vi "HideVIWindow.vi"(8 "ErrorIn":errorcluster, 11 "VIPath":path) -> (0 "ErrorOut":errorcluster)   [LabVIEW 2018]
doc: "This VI is used to Hide the inputted VIs Window. Subsequent calls to RestoreVI Window will restore the VIs Window.\n\nCopyright © 2011 Epimedia, Inc. All Rights Reserved.\n\nThe Epimedia Application Library is Copyright © 2009-2011 Epimedia, Inc. \nAll Rights Reserved. Used under license."
panel:
  # "Copyright © 2011 Epimedia, Inc. All Rights Reserved.\n\nThe Epimedia Application Library is Copyright © 2009-2011 Epimedia, Inc. \nAll Rights Reserved. Used under license."
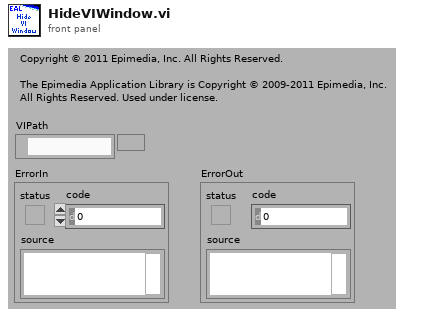
[diagram p1: front panel]
types:
  T1 = enum32{"Invalid", "Standard", "Closed", "Hidden", "Minimized", "Maximized"}
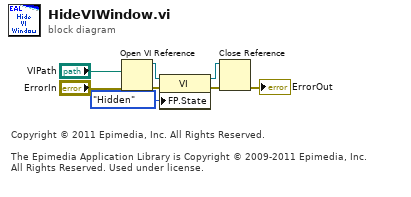
[diagram p0: block diagram]
diagram:
  # "Copyright © 2011 Epimedia, Inc. All Rights Reserved.\n\nThe Epimedia Application Library is Copyright © 2009-2011 Epimedia, Inc. \nAll Rights Reserved. Used under license."
  n1 = Open VI Reference(vi path="VIPath", error in (no error)="ErrorIn") -> (vi reference=w8:refnum<vi>, error out=w7:errorcluster)  [unwired: 4 out]
  n2 = property class="VI"(reference=w8, error in=w7, "FP.State"=T1."Hidden" ("Front Panel Window:State")) -> (reference out=w1:refnum<vi>, error out=w3:errorcluster)
  n3 = Close Reference(reference=w1, error in (no error)=w3) -> (error out=→"ErrorOut":errorcluster)
